vi "Example Callback.vi"() -> ()   [LabVIEW 2013]
uses:
  C:/tf/play/labview/Tinkerforge.dll
  Tinkerforge.dll
panel:
  out "timestamp":i64
  out "weekday":u8
  out "centisecond":u8
  out "second":u8
  out "minute":u8
  out "hour":u8
  out "month":u8
  out "day":u8
  in  "stop":bool
  out "year":i32
  in  "uid":string="abc"
  in  "port":i32=4223
  in  "host":string="localhost"
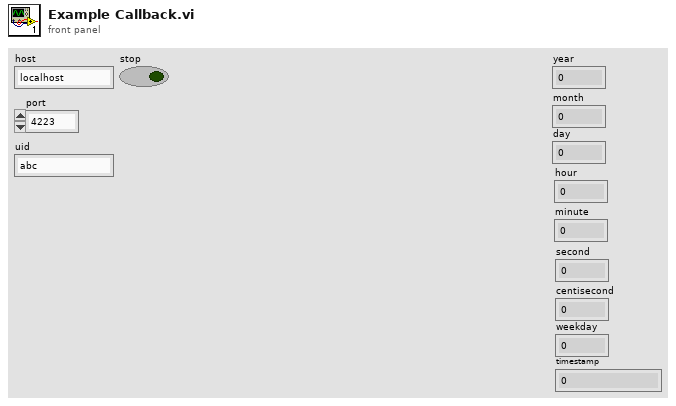
[diagram p1: front panel]
types:
  T1 = cluster{"year":i32, "month":u8, "day":u8, "hour":u8, "minute":u8, "second":u8, "centisecond":u8, "weekday":u8, "timestamp":i64}
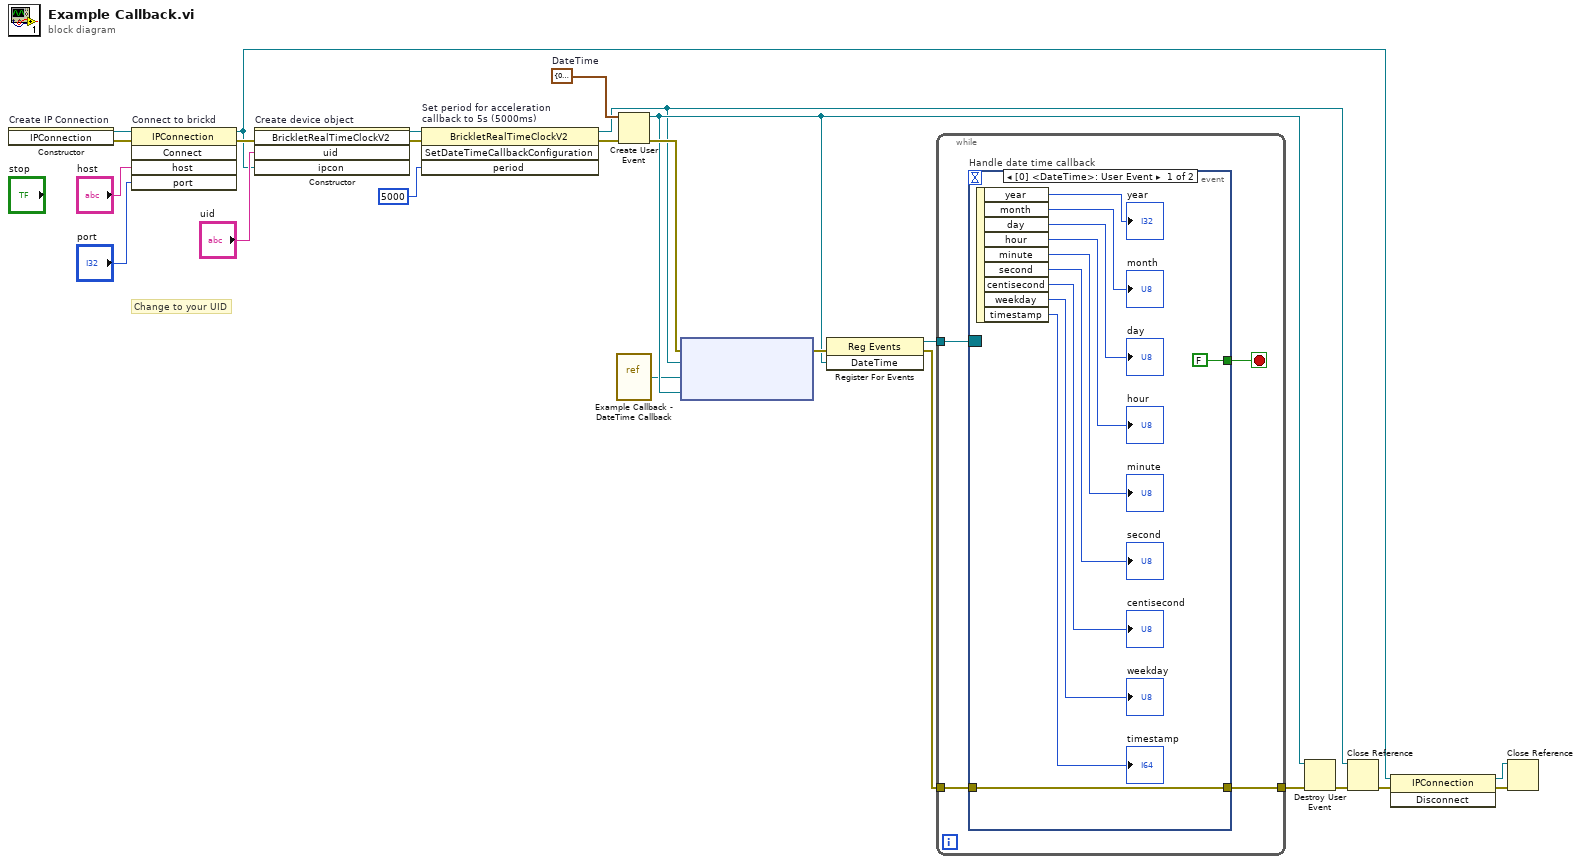
[diagram p0: block diagram]
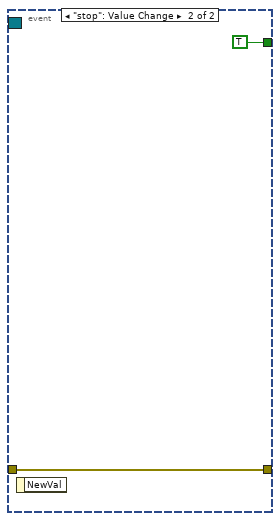
[diagram p2: hidden frame]
diagram:
  w8 = T1 {"year"=0, "month"=0, "day"=0, "hour"=0, "minute"=0, "second"=0, "centisecond"=0, "weekday"=0, "timestamp"=0}  # DateTime
  # "Change to your UID"
  n1 = constructor on="Create IP Connection" class="IPConnection"() -> (reference out=w24:refnum<k24>, error out=w2:errorcluster)  [unwired: 3 in, 1 out]
  n2 = invoke on="Connect to brickd" class="IPConnection" method="Connect"(reference=w24, error in=w2, "host"="host", "port"="port") -> (reference out=w17:refnum<k24>, error out=w20:errorcluster)  [unwired: 1 in, 3 out]
  n3 = constructor on="Create device object" class="BrickletRealTimeClockV2"(error in=w20, "uid"="uid", "ipcon"=w17) -> (reference out=w5:refnum<k24>, error out=w7:errorcluster)  [unwired: 2 in, 3 out]
  n4 = invoke on="Set period for acceleration\ncallback to 5s (5000ms)" class="BrickletRealTimeClockV2" method="SetDateTimeCallbackConfiguration"(reference=w5, error in=w7, "period"=i64 5000) -> (reference out=w4:refnum<k24>, error out=w6:errorcluster)  [unwired: 1 in, 2 out]
  n5 = vi-ref "Example Callback - DateTime Callback.vi"() -> ("vi reference"=w1:refnum<vi>)
  n6 = Create User Event(user event datatype=w8, error in=w6) -> (user event=w10:refnum<user-event>, error out=w15:errorcluster)
  n7 = node ("Register Event Callback")(w15, w4, w1, w10) -> (w14:errorcluster)  [unwired: 1 in, 1 out]
  n8 = register-events(error in=w14, w10) -> (reference out=w13:refnum<event-registration>, error out=w11:errorcluster)  [unwired: 1 in]
  n9 = while {
    tunnel: w13 -> [w28]
    tunnel: [w27] -> w12
    tunnel: w11 -> [w26]
    stop <- w25 stop-if-true
    n10 = event "Handle date time callback" shown="[0] <DateTime>: User Event" {
      selector: w28 -> [_ _]
      dyn-events: _ -> [_ _]
      timeout: _ -> [_ _]
      tunnel: [w39 w40] -> w27
      tunnel: w26 -> [w39 w40]
      tunnel: [FALSE TRUE] -> w25
      event User Event {
        n11 = event-data() -> ("year"=→"year":i32, "month"=→"month":u8, "day"=→"day":u8, "hour"=→"hour":u8, "minute"=→"minute":u8, "second"=→"second":u8, "centisecond"=→"centisecond":u8, "weekday"=→"weekday":u8, "timestamp"=→"timestamp":i64)  [unwired: 1 in]
      }
      event "stop": Value Change {
        n12 = event-data() -> ()  [unwired: 1 in, 1 out]
      }
    }
  }
  n13 = Destroy User Event(user event=w10, error in=w12) -> (error out=w9:errorcluster)
  n14 = Close Reference(reference=w4, error in (no error)=w9) -> (error out=w19:errorcluster)
  n15 = invoke class="IPConnection" method="Disconnect"(reference=w17, error in=w19) -> (reference out=w16:refnum<k24>, error out=w18:errorcluster)  [unwired: 1 in, 1 out]
  n16 = Close Reference(reference=w16, error in (no error)=w18) -> ()  [unwired: 1 out]
